vi "CMC_Using_Temperature.vi"() -> ()   [LabVIEW 2013]
doc: "This VI is designed to give experience using the Auto Tool. Refer to the LabVIEW Core I course for instructions."
panel:
  in  "Delay (sec)":dbl(slide) scale=0.0..10.0 scale format="%.1f"
  in  "Number of Measurements":i32
  out "Temperature Graph":cluster{dbl[], dbl[]}(graph)
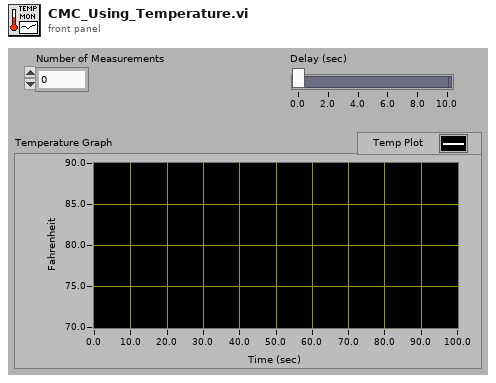
[diagram p1: front panel]
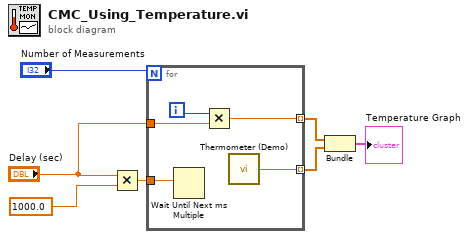
[diagram p0: block diagram]
diagram:
  n1 = Multiply(x="Delay (sec)", y=1000.0) -> (x*y=w6:dbl)
  n2 = for {
    N: "Number of Measurements" -> [_]
    tunnel: w6 -> [w12]
    tunnel: "Delay (sec)" -> [w10]
    tunnel: [w9] -> w5 mode=indexing
    tunnel: [w8] -> w4 mode=indexing
    i -> [w11]
    n3 = Wait Until Next ms Multiple(millisecond multiple=w12) -> ()  [unwired: 1 out]
    n4 = Multiply(x=w11, y=w10) -> (x*y=w9:dbl)
    n5 = call "Thermometer (Demo).vi"() -> ("Temperature"=w8:dbl)  [unwired: 1 in]
  }
  n6 = Bundle(w5, w4) -> (→"Temperature Graph":cluster{dbl[], dbl[]})  [unwired: 1 in]
